vi "Get Coordinates.vi"(8 "error in (no error)":errorcluster, 9 "Plot ID":i32, 11 "3D Pie.lvclass in":refnum<class "3D Pie.lvclass">) -> (0 "error out":errorcluster, 1 "Coordinates System":enum16{"Cartesian", "Cylindrical", "Spherical"}(ring), 3 "3D Pie.lvclass out":refnum<class "3D Pie.lvclass">)   [LabVIEW 2017, in "3D Pie.lvclass"]
uses:
  <vilib>/Math Plots/3D Math Plots/3D Pie/3D Pie/3D Pie.lvclass
  <vilib>/Math Plots/3D Math Plots/3D Pie/3D Pie/3D Pie.lvclass/3D Pie.ctl
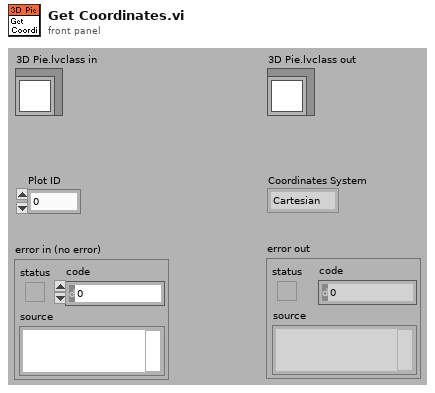
[diagram p1: front panel]
types:
  T1 = typedef "3D Pie.lvclass/3D Pie Property Array.ctl" = T2[]
  T2 = typedef "3D Pie.lvclass/3D Pie Property.ctl" = cluster{"General Property":cluster{"Plot Name":string, "Coordinate System":enum16{"Cartesian", "Cylindrical", "Spherical"}, "Opacity":sgl}, "Projection Property":cluster{"Draw XY":bool, "Draw YZ":bool, "Draw XZ":bool}, "Plot Property":cluster{"Line Style":T3, "Line Width":sgl, "Line Color":u32, "Antialiasing":bool}, "Pie Property":cluster{"Pie Height":sgl, "Pie Center":cluster{"X":sgl, "Y":sgl, "Z":sgl}, "Label Mode":enum16{"None", "Show Percentage", "Show String"}, "Label Size":u16, "Label Color":u32, "Color Pair Array":cluster{"Color":u32, "String":string}[], "Slice Offset?":bool}}
  T3 = typedef "3D Plot.lvclass/Line Type.ctl" = enum16{"None", "Solid", "Dash", "Dot", "Dash Dot"}
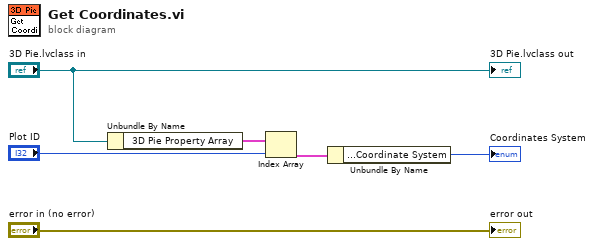
[diagram p0: block diagram]
diagram:
  n1 = Unbundle By Name("3D Pie.lvclass in") -> ("3D Pie Property Array"=w6:T1)
  n2 = Index Array(array=w6, index="Plot ID") -> (element=w5:T2)
  n3 = Unbundle By Name(w5) -> ("General Property.Coordinate System"=→"Coordinates System":enum16{"Cartesian", "Cylindrical", "Spherical"})
  "3D Pie.lvclass out" <- "3D Pie.lvclass in"
  "error out" <- "error in (no error)"
